vi "Variant to Meta Data.vi"(8 "Error In":errorcluster, 9 "Name":string, 10 "key (optional)":string, 11 "Value":variant) -> (0 "Error Out":errorcluster, 1 "Name out":string, 2 "deleted path":path, 3 "Meta data":string)   [LabVIEW 2019]
uses:
  <vilib>/Utility/config.llb/NI_LVConfig.lvlib
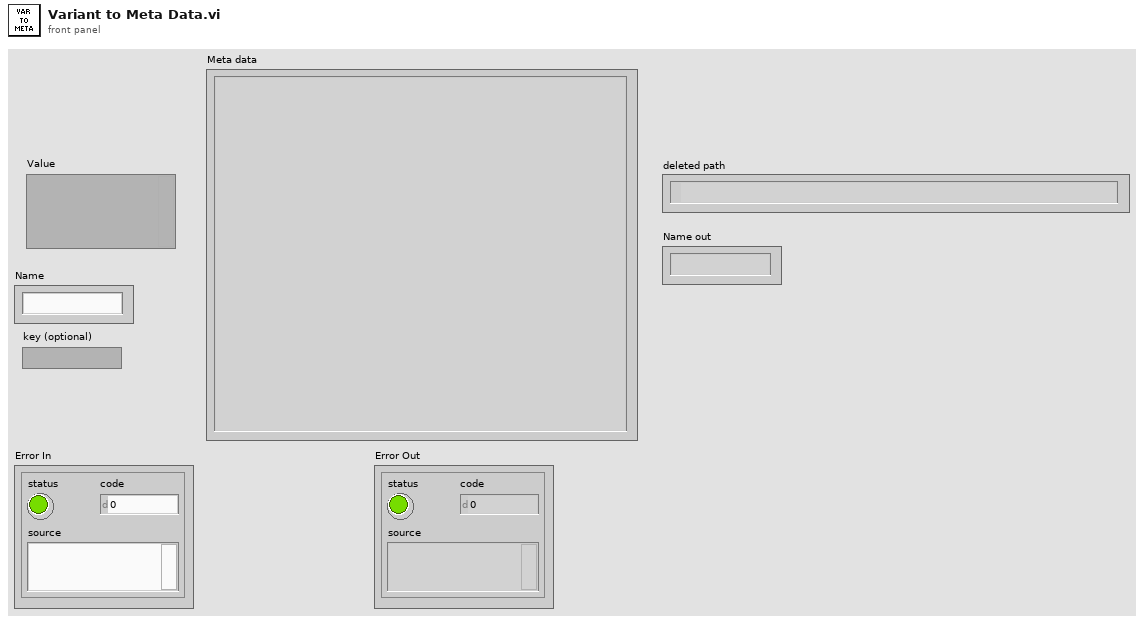
[diagram p1: front panel]
types:
  T1 = typedef "NI_LVConfig.lvlib/Config Data RefNum.ctl" = refnum<k1>
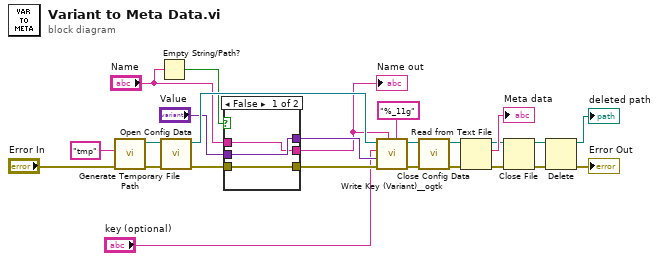
[diagram p0: block diagram]
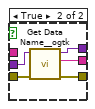
[diagram p2: hidden frame]
diagram:
  n1 = call <vilib>:"Generate Temporary File Path.vi"("error in (no error)"="Error In", "Temporary File Extension (tmp)"="tmp") -> ("error out"=w12:errorcluster, "Unique Temporary File Path"=w24:path)  [unwired: 8 in]
  n2 = Empty String/Path?(string/path="Name") -> (empty?=w8:bool)
  n3 = call <vilib>:"Open Config Data.vi"("error in (no error)"=w12, "configuration file path"=w24) -> ("error out"=w7:errorcluster, "refnum"=w23:T1)  [unwired: 7 in, 1 out]
  n4 = case shown="False" w8 {
    tunnel: "Value" -> [w28 w33]
    tunnel: [w26 w32] -> w3
    tunnel: w7 -> [w27 w31]
    tunnel: [w27 w30] -> w6
    tunnel: [w28 w29] -> w5
    tunnel: "Name" -> [w26 _]
    frame False {
    }
    frame True {
      n5 = call <userlib>:"Get Data Name__ogtk.vi"("error in (no error)"=w31, "Data"=w33) -> ("error out"=w30:errorcluster, "Data Name"=w32:string, "Data dup"=w29:variant)  [unwired: 7 in]
    }
  }
  "Name out" <- w3
  n6 = call <userlib>:"Write Key (Variant)__ogtk.vi"("float number format"="%_11g", "section"=w3, "error in (no error)"=w6, "key-value"=w5, "key (optional)"="key (optional)", "refnum"=w23) -> ("error out"=w22:errorcluster, "refnum out"=w21:T1)  [unwired: 4 in]
  n7 = call <vilib>:"Close Config Data.vi"("error in (no error)"=w22, "refnum"=w21) -> ("error out"=w19:errorcluster, "file path"=w20:path)  [unwired: 8 in]
  n8 = Read from Text File(file (use dialog)=w20, error in=w19) -> (refnum out=w17:refnum<file>, text=→"Meta data":string, error out=w16:errorcluster)  [unwired: 2 in, 1 out]
  n9 = Close File(refnum=w17, error in=w16) -> (path=w14:path, error out=w15:errorcluster)
  n10 = Delete(path (use dialog)=w14, error in=w15) -> (deleted path=→"deleted path":path, error out=→"Error Out":errorcluster)  [unwired: 3 in, 1 out]
